vi "Insert Subroutine.vi"(0 "ITest Executive in":refnum<class "ITest Executive.lvclass">, 1 "Parent ID":string, 5 "Name":string, 9 "File Path":string, 11 "error in (no error)":errorcluster, 12 "Insertion Index":i32=-1, 13 "Path Builder":refnum<class "IPath Builder.lvclass">, 14 "Persistence":refnum<class "IPersist.lvclass">) -> (3 "Unique ID out":string, 4 "ITest Executive out":refnum<class "ITest Executive.lvclass">, 8 "Replaced?":bool, 15 "error out":errorcluster)   [LabVIEW 2019, in "Test Executive.lvlib" / "ITest Executive.lvclass"]
uses:
  <vilib>/gpm_packages/@cs/test-executive/Source/Test Executive/ITestExecutive/ITest Executive.lvclass
  <vilib>/gpm_packages/@cs/persistence/source/IPersist/IPersist.lvclass
  <vilib>/gpm_packages/@cs/test-executive/Source/Path Builder/IPath Builder/IPath Builder.lvclass
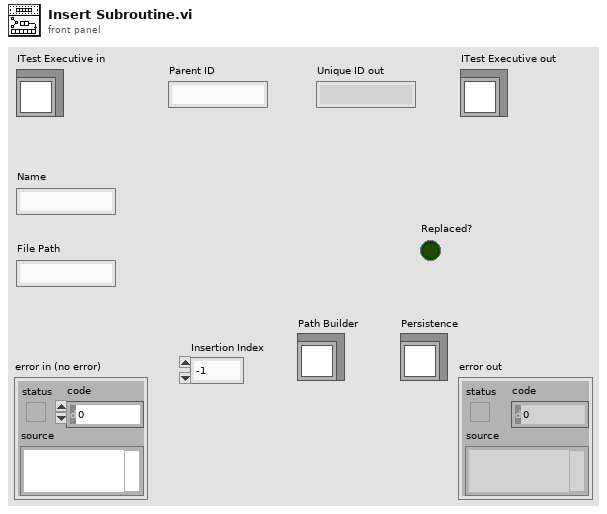
[diagram p1: front panel]
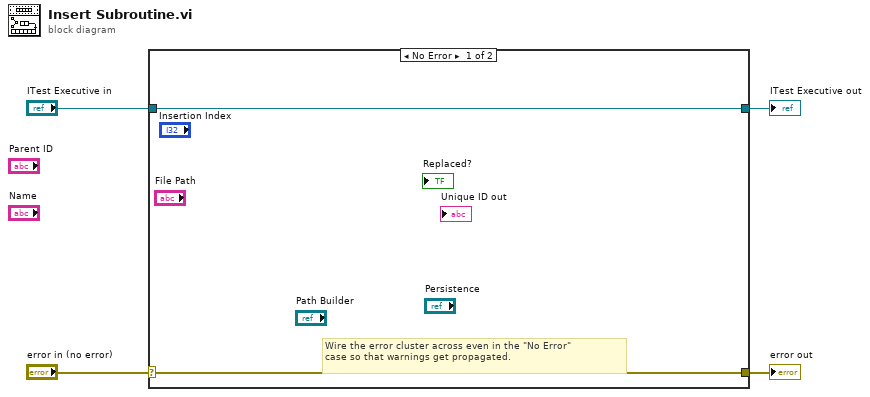
[diagram p0: block diagram]
diagram:
  n1 = case shown="No Error" "error in (no error)" {
    selector: "error in (no error)" -> [w5 w8]
    tunnel: [w5 w8] -> w3
    tunnel: [w6 w7] -> w1
    tunnel: "ITest Executive in" -> [w6 w7]
    frame No Error {
      # "Wire the error cluster across even in the \"No Error\"\ncase so that warnings get propagated."
    }
    frame Error {
    }
  }
  "error out" <- w3
  "ITest Executive out" <- w1
